vi "Test3.vi"() -> ()   [LabVIEW 2021]
panel:
  out "Intensity Graph":dbl[][](graph)
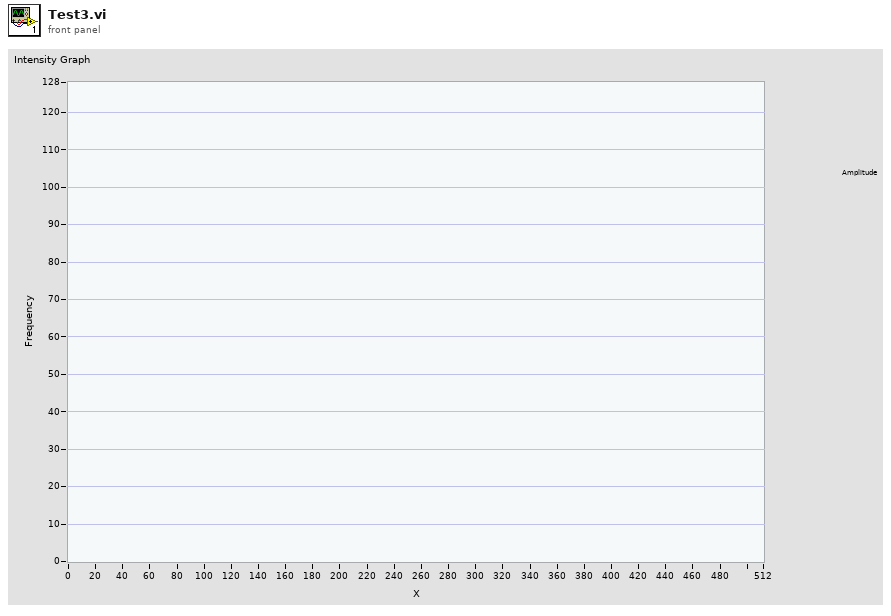
[diagram p1: front panel]
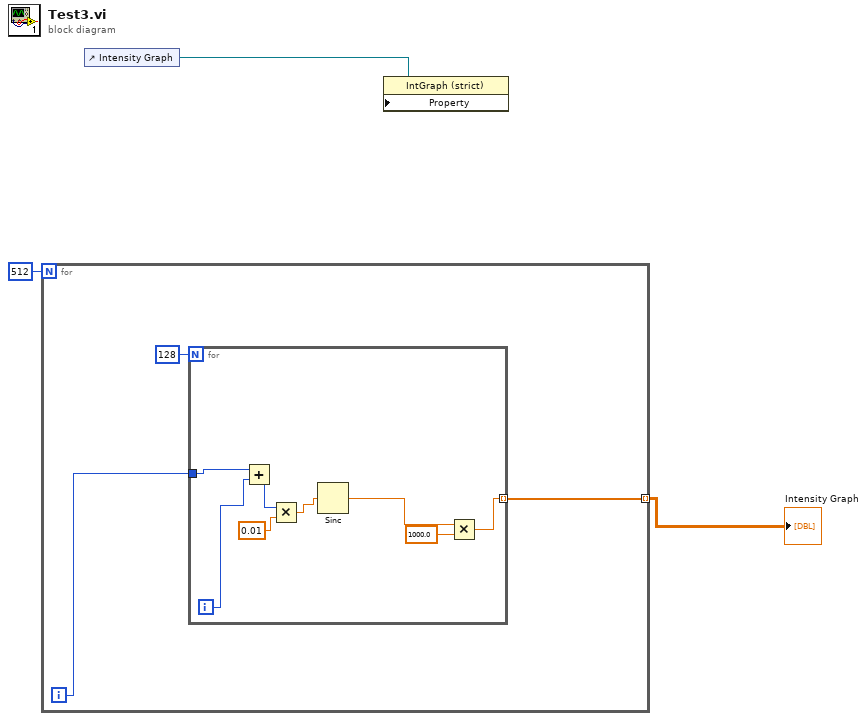
[diagram p0: block diagram]
diagram:
  n1 = for {
    N: 512 -> [_]
    tunnel: [w5] -> w2 mode=indexing
    i -> [w4]
    n2 = for {
      N: 128 -> [_]
      tunnel: [w13] -> w5 mode=indexing
      tunnel: w4 -> [w11]
      i -> [w10]
      n3 = Add(x=w11, y=w10) -> (x+y=w8:i32)
      n4 = Multiply(x=w8, y=0.01) -> (x*y=w9:dbl)
      n5 = Sinc(1:w9) -> (0:w14:dbl)
      n6 = Multiply(x=w14, y=1000.0) -> (x*y=w13:dbl)
    }
  }
  "Intensity Graph" <- w2
  n7 = control-ref of="Intensity Graph"() -> (w1:refnum<vi>)
  n8 = property class="IntGraph (strict)" props=[](reference=w1) -> ()  [unwired: 2 in, 2 out]
